vi "Clear All Faults.vi"(8 "error in (no error)":errorcluster, 11 "target address (localhost)":string="localhost") -> (0 "error out":errorcluster)   [LabVIEW 2020]
doc: "Clears all active faults on the target."
uses:
  <resource>/objmgr/ni.var.rc
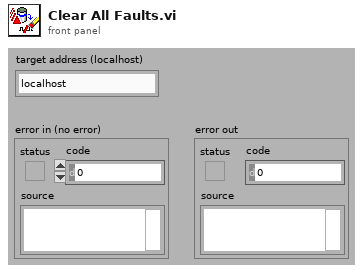
[diagram p1: front panel]
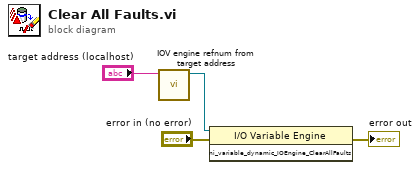
[diagram p0: block diagram]
diagram:
  n1 = call <vilib>:"IOV engine refnum from target address.vi"("target address"="target address (localhost)") -> ("reference out"=w2:refnum<k21>)  [unwired: 10 in]
  n2 = invoke class="I/O Variable Engine" method="ni_variable_dynamic_IOEngine_ClearAllFaults"(reference=w2, error in="error in (no error)") -> (error out=→"error out":errorcluster)  [unwired: 1 in, 2 out]
